vi "test Pointer Is Valid Checks.vi"(8 "error in (no error)":errorcluster, 11 "TestCase in":refnum<class "Memory Manager Tests.lvclass">) -> (0 "error out":errorcluster, 3 "TestCase out":refnum<class "Memory Manager Tests.lvclass">)   [LabVIEW 2020, in "Memory Manager Tests.lvclass"]
uses:
  Memory Manager Tests.lvclass
  <vilib>/Utility/file.llb/Application Directory.vi
  <vilib>/Utility/libraryn.llb/Check if File or Folder Exists.vi
  <vilib>/addons/_JKI Toolkits/VI Tester/TestCase.llb/TestCase.lvclass
  C:/Program Files/National Instruments/LabVIEW 2020/vi.lib/addons/_JKI Toolkits/VI Tester/TestCase.llb/TestCase.lvclass
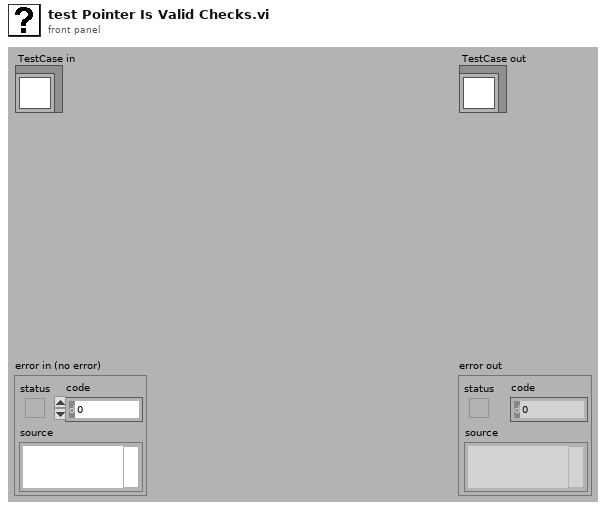
[diagram p1: front panel]
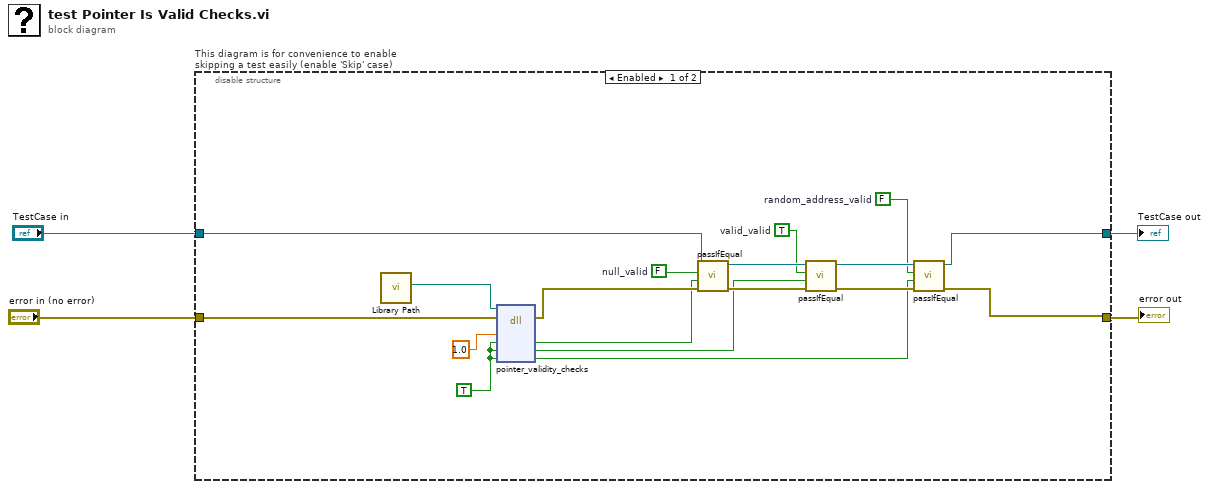
[diagram p0: block diagram]
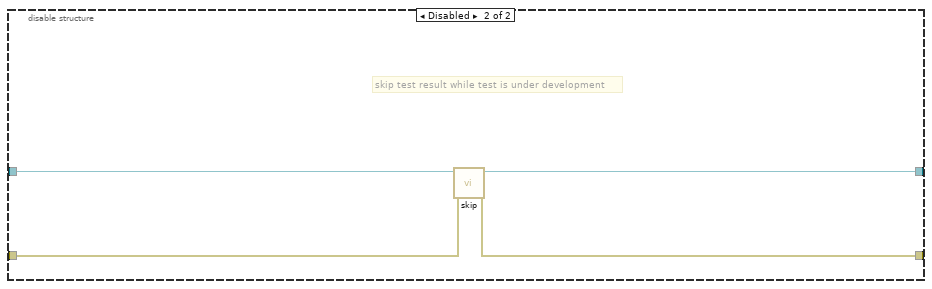
[diagram p2: hidden frame]
diagram:
  n1 = disable-structure "This diagram is for convenience to enable skipping a test easily (enable 'Skip' case)" shown="Enabled" {
    disable-tunnel: "TestCase in" -> [w22 w26]
    disable-tunnel: [w15 w24] -> w1
    disable-tunnel: [w16 w25] -> w3
    disable-tunnel: "error in (no error)" -> [w19 w23]
    frame Enabled {
      w6 = FALSE  # null_valid
      w7 = TRUE  # valid_valid
      w8 = FALSE  # random_address_valid
      w17 = TRUE
      n2 = call "Library Path.vi"() -> ("Library Path"=w20:path)  [unwired: 11 in]
      n3 = dll-call lib="C:/Users/JamesMcNally/Documents/RustInterop/Rust-LabVIEW-Interop/target/debug/labview_test_library.dll" fn="pointer_validity_checks"(path in=w20, error in=w19, "valid_pointer"=1.0, "null_valid"=w17, "valid_valid"=w17, "random_address_valid"=w17) -> (error out=w18:errorcluster, "null_valid"=w11:bool, "valid_valid"=w10:bool, "random_address_valid"=w9:bool)  [unwired: 3 in, 1 out]
      n4 = call-dynamic "passIfEqual.vi"("error in (no error)"=w18, "y"=w11, "x"=w6, "TestCase in"=w22) -> ("error out"=w21:errorcluster, "TestCase out"=w13:refnum<class "Memory Manager Tests.lvclass">)  [unwired: 6 in]
      n5 = call-dynamic "passIfEqual.vi"("error in (no error)"=w21, "y"=w10, "x"=w7, "TestCase in"=w13) -> ("error out"=w14:errorcluster, "TestCase out"=w12:refnum<class "Memory Manager Tests.lvclass">)  [unwired: 6 in]
      n6 = call-dynamic "passIfEqual.vi"("error in (no error)"=w14, "y"=w9, "x"=w8, "TestCase in"=w12) -> ("error out"=w16:errorcluster, "TestCase out"=w15:refnum<class "Memory Manager Tests.lvclass">)  [unwired: 6 in]
    }
    frame Disabled {
      # "skip test result while test is under development"
      n7 = call <vilib>:"skip.vi"("error in (no error)"=w23, "TestCase in"=w26) -> ("error out"=w25:errorcluster, "TestCase out"=w24:refnum<class "Memory Manager Tests.lvclass">)  [unwired: 8 in]
    }
  }
  "error out" <- w3
  "TestCase out" <- w1
